vi "Process.vi"(8 "error in":errorcluster, 11 "Logger":refnum<class "Logger.DSC.lvclass">) -> (0 "error out":errorcluster, 3 "Logger out":refnum<class "Logger.DSC.lvclass">)   [LabVIEW 2016, in "Logger.DSC.lvclass"]
doc: "---------------------------------------------------------------\nJKI State Machine Objects™\nhttp://jki.net/state-machine-objects/\nCopyright (C) 2005-2015, JKI <info@jki.net>\nALL RIGHTS RESERVED"
uses:
  Logger.DSC.lvclass
  C:/Program Files (x86)/National Instruments/LabVIEW 2016/vi.lib/JKI/JKI SMO/SMO/SMO.lvclass
  <vilib>/JKI/JKI SMO/SMO/Typedefs/Parent Call--Enum.ctl
  <vilib>/JKI/JKI SMO/SMO/SMO.lvclass
  <resource>/objmgr/ni.var.rc
panel:
  out "Writable":bool
  out "URL":string
  out "Readable":bool
  out "Parent":refnum<k21>
  out "Name":string
  out "Engine":refnum<k21>
  out "Class Identifier":string
  # "For instructions on how to use the JKI State Machine Objects, examples and video tutorials, visit:\nhttp://jki.net/state-machine-objects/\n\nJKI State Machine Objects™\nhttp://jki.net/state-machine-objects/\nCopyright (C) 2005-2015, JKI <info@jki.net>\nALL RIGHTS RESERVED"
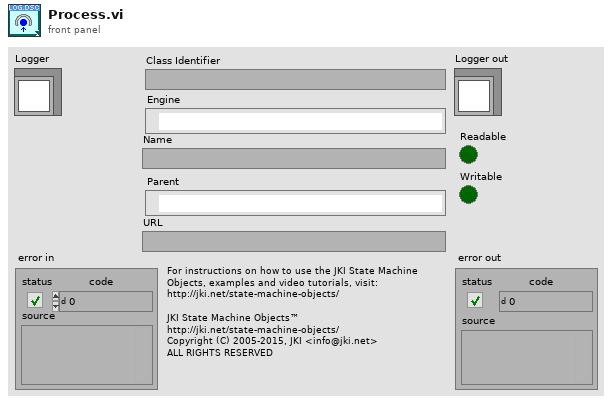
[diagram p1: front panel]
types:
  T1 = typedef "SMO.lvclass/Parent Call--Enum.ctl" = enum16{"Allows parent to run", "Does not request parent to run"}
  T2 = enum32{"invalid app kind", "Development System", "Run Time System", "Student Edition", "Embedded LabVIEW", "Evaluation", "Custom"}
  T3 = enum32{"Invalid", "Standard", "Closed", "Hidden", "Minimized", "Maximized"}
  T4 = enum32{"Bad", "Idle", "Run top level", "Running"}
  T5 = cluster{"Core":cluster{"Current VI Reference":refnum<vi>, "Close Panel on Exit?":bool, "error":errorcluster}, "Self Reference":refnum<class "Logger.DSC.lvclass">, "shared variable address":string, "data in":variant, "data out":variant}
  T6 = cluster{"Current VI Reference":refnum<vi>, "Close Panel on Exit?":bool, "error":errorcluster}
  T7 = typedef "SMO.lvclass/Protected Events.ctl" = cluster{"StopProcesses":refnum<user-event>, "AbortProcesses":refnum<user-event>, "Config Changed":refnum<user-event>, "Dependency":refnum<user-event>}
  T8 = typedef "Logger.DSC.lvclass/PrivateEvents--Cluster.ctl" = cluster{"Set Address":refnum<user-event>, "Write Variable":refnum<user-event>}
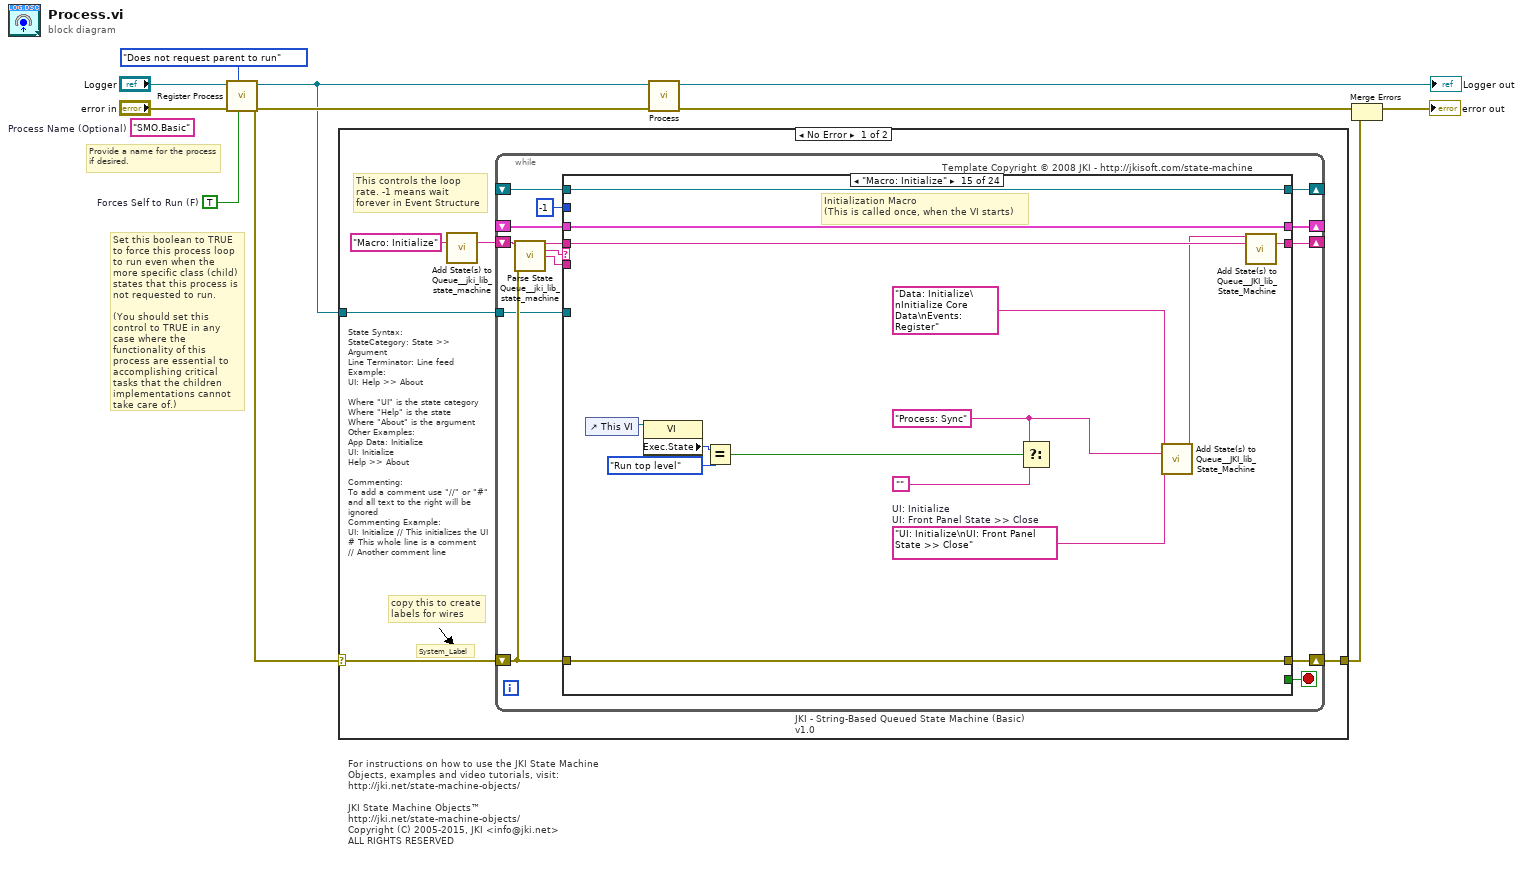
[diagram p0: block diagram]
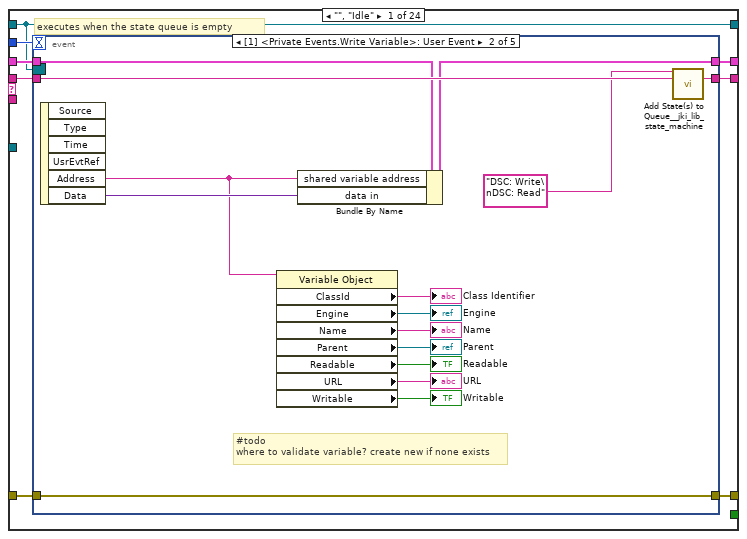
[diagram p2: hidden frame]
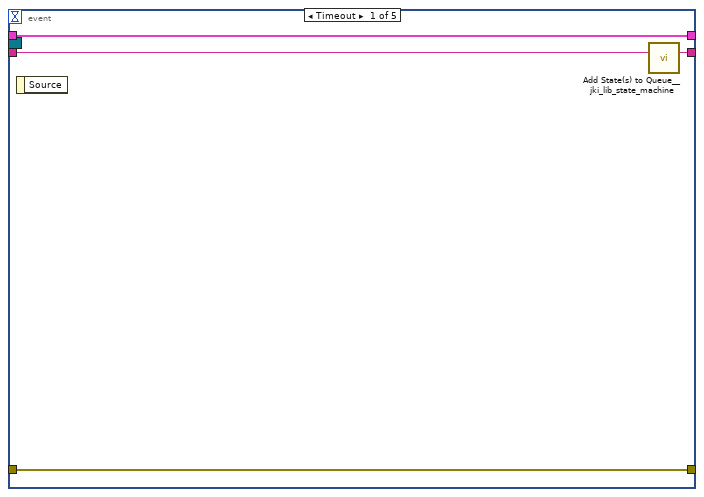
[diagram p3: hidden frame]
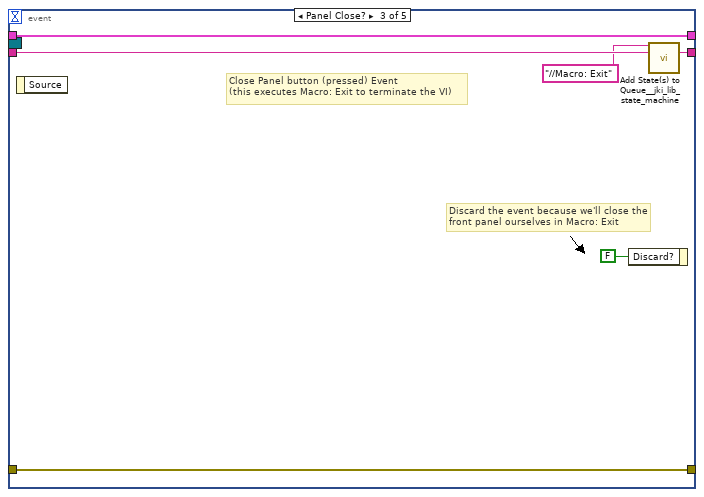
[diagram p4: hidden frame]
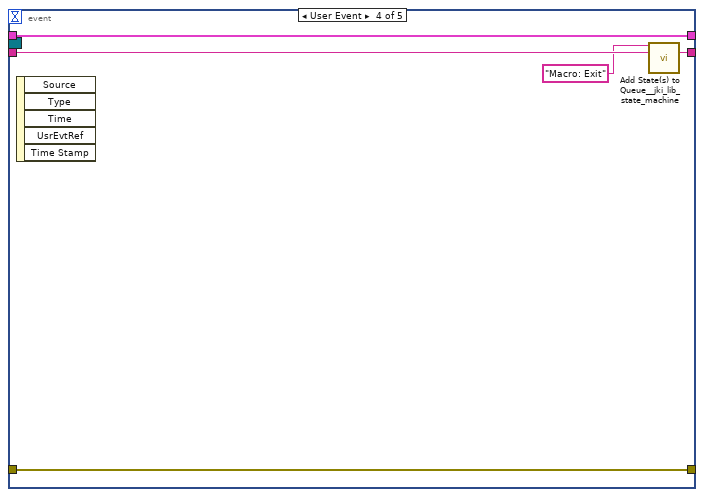
[diagram p5: hidden frame]
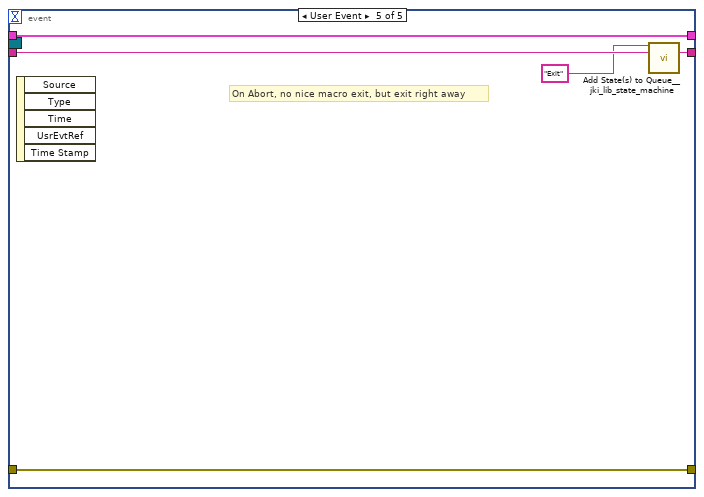
[diagram p6: hidden frame]
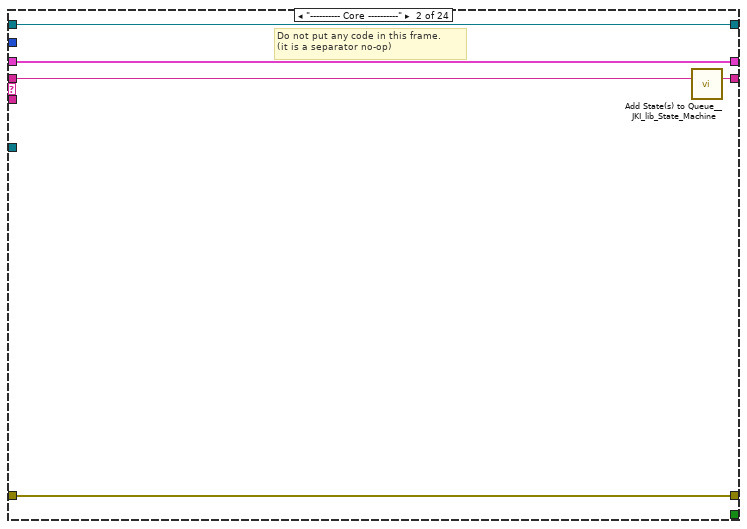
[diagram p7: hidden frame]
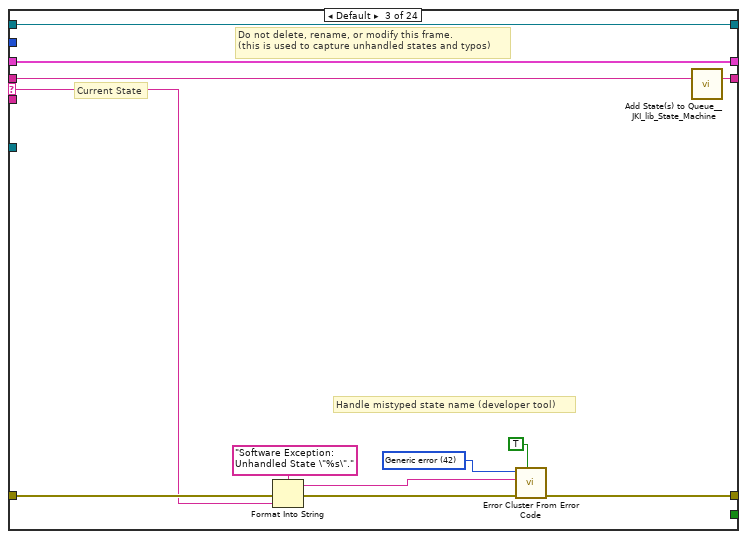
[diagram p8: hidden frame]
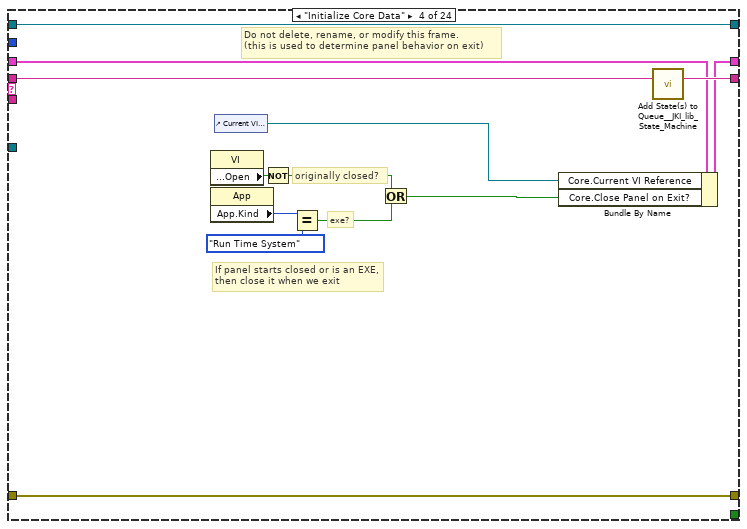
[diagram p9: hidden frame]
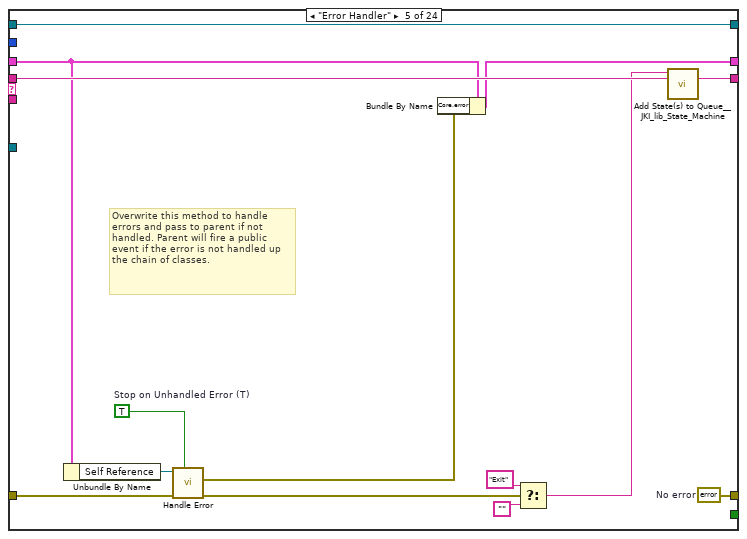
[diagram p10: hidden frame]
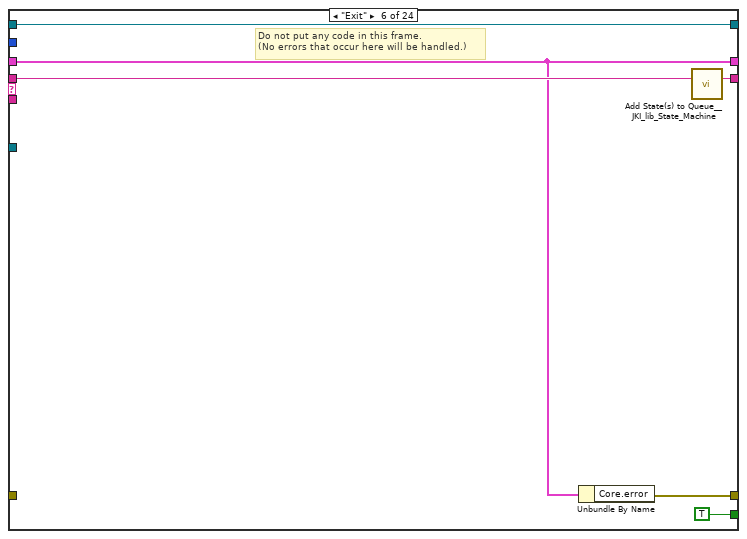
[diagram p11: hidden frame]
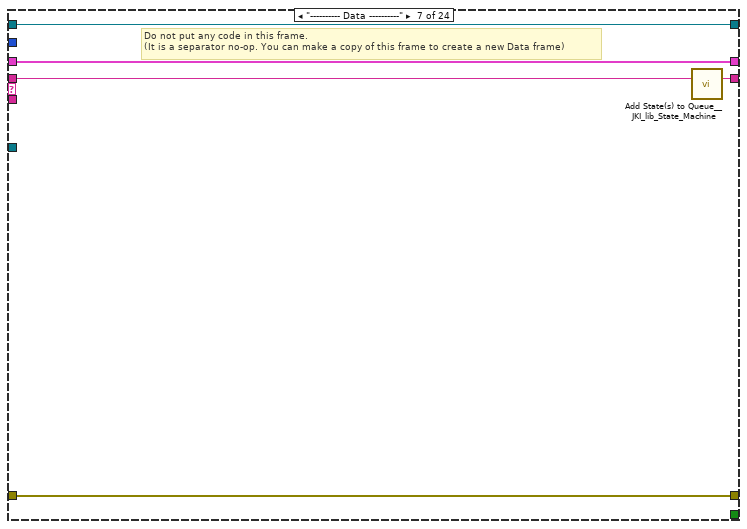
[diagram p12: hidden frame]
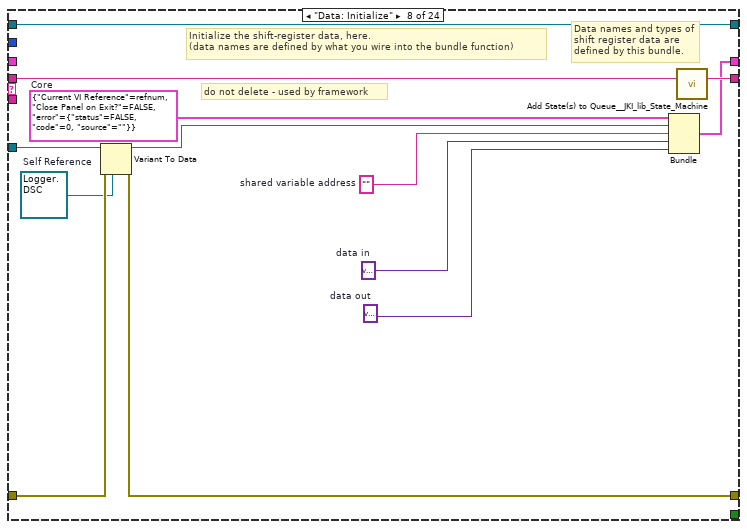
[diagram p13: hidden frame]
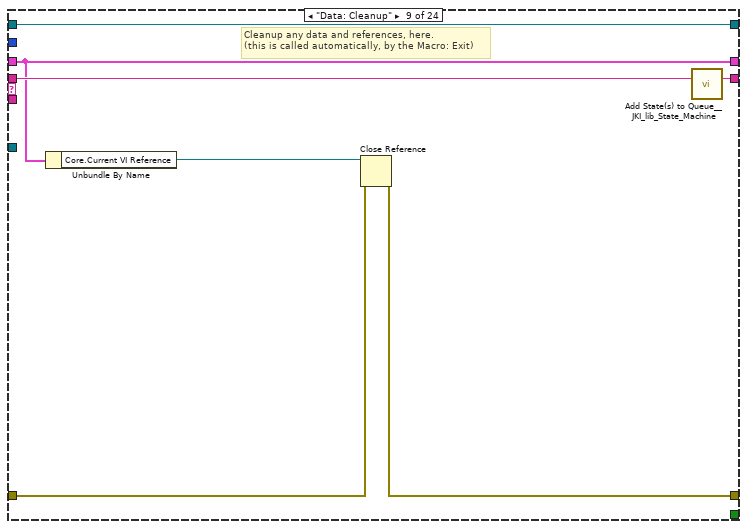
[diagram p14: hidden frame]
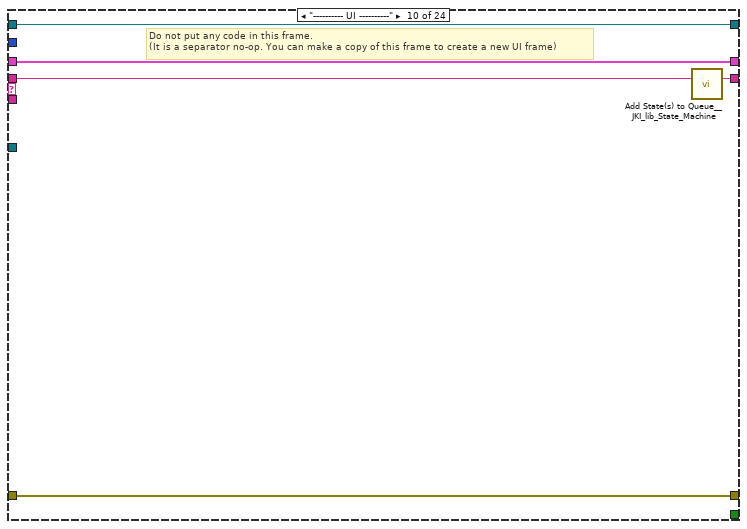
[diagram p15: hidden frame]
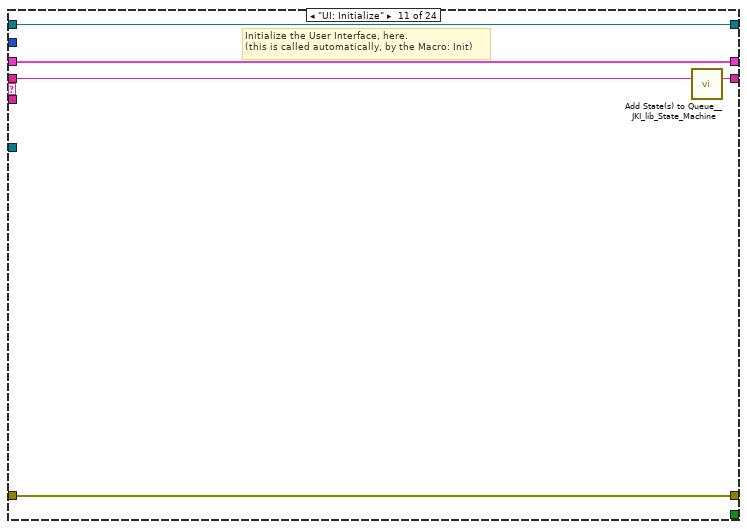
[diagram p16: hidden frame]
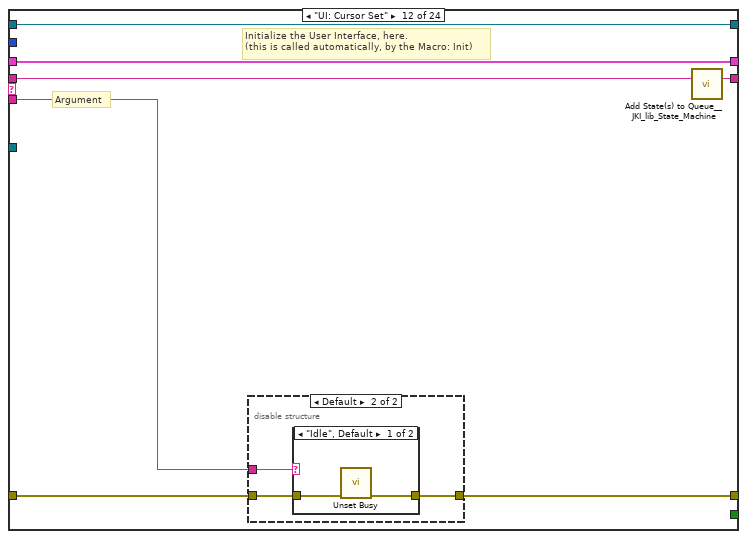
[diagram p17: hidden frame]
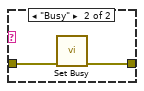
[diagram p19: hidden frame]
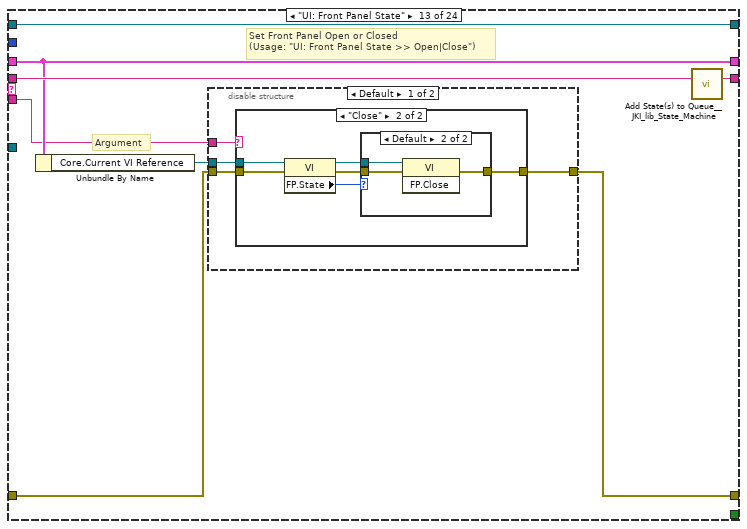
[diagram p20: hidden frame]
diagram:
  w1 = TRUE  # Forces Self to Run (F)
  (unwired) "SMO.Basic"  # Process Name (Optional)
  # "Provide a name for the process\nif desired."
  # "Set this boolean to TRUE to force this process loop to run even when the more specific class (child) states that this process is not requested to run.\n\n(You should set this control to TRUE in any case where the functionality of this process are essential to accomplishing critical tasks that the children implementations cannot take care of.)"
  # "For instructions on how to use the JKI State Machine Objects, examples and video tutorials, visit:\nhttp://jki.net/state-machine-objects/\n\nJKI State Machine Objects™\nhttp://jki.net/state-machine-objects/\nCopyright (C) 2005-2015, JKI <info@jki.net>\nALL RIGHTS RESERVED"
  n1 = call <vilib>:"Register Process.vi"("Forces Self to Run (F)"=w1, "Parent Call"=Parent_Call--Enum."Does not request parent to run", "error in (no error)"="error in", "SMO"="Logger") -> ("error out"=w7:errorcluster, "SMO out"=w6:refnum<class "Logger.DSC.lvclass">)  [unwired: 6 in]
  n2 = case shown="No Error" w7 {
    selector: w7 -> [w12 w308]
    tunnel: w6 -> [w13 _]
    tunnel: [w11 w308] -> w3
    frame No Error {
      # "State Syntax:\nStateCategory: State >> Argument\nLine Terminator: Line feed\nExample:\nUI: Help >> About\n\nWhere \"UI\" is the state category\nWhere \"Help\" is the state\nWhere \"About\" is the argument\nOther Examples:\nApp Data: Initialize\nUI: Initialize\nHelp >> About\n\nCommenting:\nTo add a comment use \"//\" or \"#\" and all text to the right will be ignored\nCommenting Example:\nUI: Initialize // This initializes the UI\n# This whole line is a comment\n// Another comment line"
      # "copy this to create labels for wires"
      # "This controls the loop rate. -1 means wait forever in Event Structure"
      # "System_Label"
      n3 = call <vilib>:"Add State(s) to Queue__jki_lib_state_machine.vi"("State(s) in (\"\")"="Macro: Initialize") -> ("States Out"=w15:string)  [unwired: 14 in]
      n4 = while "JKI - String-Based Queued State Machine (Basic) v1.0" {
        shift-right: [w22] -> _
        shift-left: _ -> [w21]
        shift-right: [w25] -> w11
        shift-left: w12 -> [w19]
        shift-right: [w24] -> _
        shift-left: w15 -> [w26]
        tunnel: w13 -> [w18]
        shift-right: [w17] -> _
        shift-left: _ -> [w16]
        stop <- w23 stop-if-true
        # "Template Copyright © 2008 JKI - http://jkisoft.com/state-machine"
        n5 = call <vilib>:"Parse State Queue__jki_lib_state_machine.vi"("State Queue"=w26, "Error In (no error)"=w19) -> ("Remaining States"=w28:string, "Current State"=w29:string, "Arguments"=w27:string)  [unwired: 11 in]
        n6 = case shown="\"Macro: Initialize\"" w29 {
          selector: w29 -> [_ _ w79 _ _ _ _ _ _ _ _ _ _ _ _ _ _ _ _ _ _ _ _ _]
          tunnel: w28 -> [w37 w77 w83 w102 w116 w122 w127 w140 w147 w152 w157 w164 w180 w212 w226 w240 w245 w256 w261 w274 w280 w285 w295 w307]
          tunnel: w27 -> [_ _ _ _ _ _ _ _ _ _ _ w158 w174 _ _ _ _ _ _ _ _ _ _ _]
          tunnel: w21 -> [w35 w74 w81 w93 w110 w118 w124 _ w142 w149 w155 w162 w176 w209 w222 w231 w242 w253 w258 w272 w278 w283 w291 w302]
          tunnel: [w34 w75 w85 w99 w111 w117 w125 w136 w143 w150 w154 w159 w177 w210 w224 w238 w243 w247 w259 w267 w276 w281 w292 w297] -> w25
          tunnel: w19 -> [w33 w75 w84 w99 w112 _ w125 w137 w144 w150 w154 w160 w178 w210 w224 w238 w243 w248 w259 w268 w276 w281 w287 w298]
          tunnel: [w36 w76 w82 w101 w115 w121 w126 w139 w146 w151 w156 w163 w179 w211 w225 w239 w244 w255 w260 w273 w279 w284 w294 w306] -> w24
          tunnel: [_ _ _ _ _ TRUE _ _ _ _ _ _ _ _ _ _ _ _ _ _ _ _ _ _] -> w23
          tunnel: [w32 w74 w81 w100 w109 w118 w124 w138 w142 w149 w155 w162 w176 w209 w222 w231 w242 w253 w258 w272 w278 w283 w291 w302] -> w22
          tunnel: -1 ("Timeout") -> [w31 _ _ _ _ _ _ _ _ _ _ _ _ _ _ _ _ _ _ _ _ _ _ _]
          tunnel: w18 -> [_ _ _ _ _ _ _ w134 _ _ _ _ _ _ _ _ _ _ _ _ _ _ _ _]
          tunnel: [w30 w73 w78 w90 w114 w119 w123 w132 w141 w148 w153 w161 w173 w208 w223 w232 w241 w254 w257 w271 w277 w282 w293 w305] -> w17
          tunnel: w16 -> [w30 w73 w78 w90 w114 w119 w123 w132 w141 w148 w153 w161 w173 w208 w223 w232 w241 w254 w257 _ w277 w282 w293 w305]
          frame "", "Idle" {
            # "executes when the state queue is empty"
            n7 = event shown="[1] <Private Events.Write Variable>: User Event" {
              selector: w30 -> [_ _ _ _ _]
              dyn-events: _ -> [_ _ _ _ _]
              timeout: w31 -> [_ _ _ _ _]
              tunnel: w37 -> [w41 w56 w62 w67 w72]
              tunnel: [w40 w55 w61 w66 w71] -> w36
              tunnel: w35 -> [w39 w53 w59 w64 w69]
              tunnel: [w38 w54 w60 w65 w70] -> w34
              tunnel: w33 -> [w38 w54 w60 w65 w70]
              tunnel: [w39 w52 w59 w64 w69] -> w32
              event Timeout {
                n8 = event-data() -> ()  [unwired: 1 in, 1 out]
                n9 = call <vilib>:"Add State(s) to Queue__jki_lib_state_machine.vi"("State(s) in (\"\")"=w41) -> ("States Out"=w40:string)  [unwired: 14 in]
              }
              event User Event {
                # "#todo\nwhere to validate variable? create new if none exists"
                n10 = event-data() -> ("Address"=w42:string, "Data"=w50:variant)  [unwired: 1 in, 4 out]
                n11 = property class="Variable Object"(reference=w42) -> ("ClassId"=→"Class Identifier":string, "Engine"=→"Engine":refnum<k21>, "Name"=→"Name":string, "Parent"=→"Parent":refnum<k21>, "Readable"=→"Readable":bool, "URL"=→"URL":string, "Writable"=→"Writable":bool)  [unwired: 1 in, 2 out]
                n12 = Bundle By Name(cluster=w53, "shared variable address"=w42, "data in"=w50) -> (w52:T5)
                n13 = call <vilib>:"Add State(s) to Queue__jki_lib_state_machine.vi"("State(s) in Front (\"\")"="DSC: Write\nDSC: Read" ("State(s) in Front (\"\")"), "State(s) in (\"\")"=w56) -> ("States Out"=w55:string)  [unwired: 13 in]
              }
              event Panel Close? {
                # "Discard the event because we'll close the front panel ourselves in Macro: Exit"
                # "Close Panel button (pressed) Event\n(this executes Macro: Exit to terminate the VI)"
                n14 = event-data() -> ()  [unwired: 1 in, 1 out]
                n15 = event-data("Discard?"=FALSE) -> ()  [unwired: 1 in, 1 out]
                n16 = call <vilib>:"Add State(s) to Queue__jki_lib_state_machine.vi"("State(s) in Front (\"\")"="//Macro: Exit", "State(s) in (\"\")"=w62) -> ("States Out"=w61:string)  [unwired: 13 in]
              }
              event User Event {
                n17 = event-data() -> ()  [unwired: 1 in, 5 out]
                n18 = call <vilib>:"Add State(s) to Queue__jki_lib_state_machine.vi"("State(s) in Front (\"\")"="Macro: Exit", "State(s) in (\"\")"=w67) -> ("States Out"=w66:string)  [unwired: 13 in]
              }
              event User Event {
                # "On Abort, no nice macro exit, but exit right away"
                n19 = event-data() -> ()  [unwired: 1 in, 5 out]
                n20 = call <vilib>:"Add State(s) to Queue__jki_lib_state_machine.vi"("State(s) in Front (\"\")"="Exit", "State(s) in (\"\")"=w72) -> ("States Out"=w71:string)  [unwired: 13 in]
              }
            }
          }
          frame "---------- Core ----------" {
            # "Do not put any code in this frame.\n(it is a separator no-op)"
            n21 = call <vilib>:"Add State(s) to Queue__JKI_lib_State_Machine.vi"("State(s) in (\"\")"=w77) -> ("States Out"=w76:string)  [unwired: 14 in]
          }
          frame Default {
            w88 = 42 items=["No error", "Argument error", "Memory is full", "Out of zone", "End of file", "File already open", "Generic file I/O error", "File not found", "File permission error", "Disk is full", "Duplicate path", "Too many files open", "System feature not enabled", "Resource file not found", "Cannot add resource", "Resource not found", "Image not found", "Image memory error", "Pen does not exist", "Config type invalid", "Config token not found", "Config parse error", "Config memory error", "Bad external code format", "Bad external code offset", "External code not present", "Null window", "Destroy window error", "Null menu", "Print aborted", "Bad print record", "Print driver error", "Windows error during printing", "Memory error during printing", "Print dialog error", "Generic print error", "Invalid device refnum", "Device not found", "Device parameter error", "Device unit error", "Cannot open device", "Device call aborted", "Generic error", "Cancelled by user", "Object ID too low", "Object ID too high", "Object not in heap", "Unknown heap", "Unknown object (invalid DefProc)", "Unknown object (DefProc not in table)", "Message out of range", "Invalid (null) method", "Unknown message", "Manager call not supported", "Bad address", "Network operation in progress", "Network operation timed out", "Connection is busy", "Network attribute not supported", "Network error", "Address in use", "System out of memory", "Connection aborted", "Connection refused", "Not connected", "Already connected", "Connection closed", "Initialization error (interapplication manager)", "Bad occurrence", "Wait on unbound occurrence handler", "Occurrence queue overflow", "Datalog type conflict", "Unused", "Unrecognized type (interapplication manager)", "Memory corrupt", "Failed to make temporary DLL", "Old CIN version", "Drag socket not found", "Failed to load drop-object", "Failed to register OLE object", "Failed to release OLE object", "Format specifier type mismatch", "Unknown format specifier", "Too few format specifiers", "Too many format specifiers", "Scan failed", "Newer CIN version", "Error converting to variant", "Runtime menu error", "Password tampered", "Variant attribute not found", "Incompatible variant data type", "Event data is not available", "Event Store is not present", "Occurrence is not found", "Event Queue is not created", "Event info is not available", "Refnum passed is NULL", "Error retrieving Class GUID", "Error retrieving CoClass GUID", "Error retrieving TypeLib GUID.", "Bad built application magic bytes.", "Specific driver is different from the specific driver associated with the Logical Name.", "There is no session opened to the class driver.", "Max Error", "MAX - Error with config objects", "MAX - Error loading configuration", "MAX - Group not supported"]
            # "Current State"
            # "Do not delete, rename, or modify this frame.\n(this is used to capture unhandled states and typos)"
            # "Handle mistyped state name (developer tool)"
            n22 = Format Into String(format string="Software Exception: Unhandled State \"%s\"." ("message"), error in=w84, w79) -> (resulting string=w87:string, error out=w86:errorcluster)  [unwired: 1 in]
            n23 = call <vilib>:"Error Cluster From Error Code.vi"("show call chain? (False)"=TRUE, "error in (no error)"=w86, "error message (\"\")"=w87, "error code (0)"=w88) -> ("error out"=w85:errorcluster)  [unwired: 5 in]
            n24 = call <vilib>:"Add State(s) to Queue__JKI_lib_State_Machine.vi"("State(s) in (\"\")"=w83) -> ("States Out"=w82:string)  [unwired: 14 in]
          }
          frame "Initialize Core Data" {
            # "Do not delete, rename, or modify this frame.\n(this is used to determine panel behavior on exit)"
            # "originally closed?"
            # "exe?"
            # "If panel starts closed or is an EXE, then close it when we exit"
            n25 = property class="VI"() -> ("Front Panel.Open"=w98:bool)  [unwired: 2 in, 2 out]
            n26 = property class="App"() -> ("App.Kind"=w97:T2)  [unwired: 2 in, 2 out]
            n27 = control-ref of="Current VI Reference"() -> (w91:refnum<vi>)
            n28 = Not(x=w98) -> (.not. x?=w95:bool)
            n29 = Equal?(x=w97, y=T2."Run Time System" ("Application:Kind")) -> (x = y?=w94:bool)
            n30 = Or(x=w95, y=w94) -> (x .or. y?=w92:bool)
            n31 = Bundle By Name(cluster=w93, "Core.Current VI Reference"=w91, "Core.Close Panel on Exit?"=w92) -> (w100:T5)
            n32 = call <vilib>:"Add State(s) to Queue__JKI_lib_State_Machine.vi"("State(s) in (\"\")"=w102) -> ("States Out"=w101:string)  [unwired: 14 in]
          }
          frame "Error Handler" {
            w103 = TRUE  # Stop on Unhandled Error (T)
            w111 = errorcluster {"status"=FALSE, "code"=0, "source"=""}  # No error
            # "Overwrite this method to handle errors and pass to parent if not handled. Parent will fire a public event if the error is not handled up the chain of classes."
            n33 = Unbundle By Name(w110) -> ("Self Reference"=w113:refnum<class "Logger.DSC.lvclass">)
            n34 = call-dynamic "Handle Error.vi"("Stop on Unhandled Error (T)"=w103, "error in"=w112, "SMO"=w113) -> ("handling error"=w104:errorcluster, "Unhandled error"=w107:errorcluster)  [unwired: 6 in, 1 out]
            n35 = Bundle By Name(cluster=w110, "Core.error"=w107) -> (w109:T5)
            n36 = Select(t="Exit", s=w104, f="") -> (s? t:f=w108:string)
            n37 = call <vilib>:"Add State(s) to Queue__JKI_lib_State_Machine.vi"("State(s) in Front (\"\")"=w108, "State(s) in (\"\")"=w116) -> ("States Out"=w115:string)  [unwired: 13 in]
          }
          frame "Exit" {
            # "Do not put any code in this frame.\n(No errors that occur here will be handled.)"
            n38 = Unbundle By Name(w118) -> ("Core.error"=w117:errorcluster)
            n39 = call <vilib>:"Add State(s) to Queue__JKI_lib_State_Machine.vi"("State(s) in (\"\")"=w122) -> ("States Out"=w121:string)  [unwired: 14 in]
          }
          frame "---------- Data ----------" {
            # "Do not put any code in this frame.\n(It is a separator no-op. You can make a copy of this frame to create a new Data frame)"
            n40 = call <vilib>:"Add State(s) to Queue__JKI_lib_State_Machine.vi"("State(s) in (\"\")"=w127) -> ("States Out"=w126:string)  [unwired: 14 in]
          }
          frame "Data: Initialize" {
            w128 = variant  # data out
            w129 = variant  # data in
            w130 = ""  # shared variable address
            w131 = T6 {"Current VI Reference"=refnum, "Close Panel on Exit?"=FALSE, "error"={"status"=FALSE, "code"=0, "source"=""}}  # Core
            w135 = refnum<class "Logger.DSC.lvclass"> refnum  # Self Reference
            # "do not delete - used by framework"
            # "Data names and types of shift register data are defined by this bundle."
            # "Initialize the shift-register data, here.\n(data names are defined by what you wire into the bundle function)"
            n41 = Variant To Data(error in=w137, type=w135, Variant=w134) -> (data=w133:refnum<class "Logger.DSC.lvclass">, error out=w136:errorcluster)
            n42 = Bundle("Core"=w131, "Self Reference"=w133, "shared variable address"=w130, "data in"=w129, "data out"=w128) -> (w138:T5)  [unwired: 1 in]
            n43 = call <vilib>:"Add State(s) to Queue__JKI_lib_State_Machine.vi"("State(s) in (\"\")"=w140) -> ("States Out"=w139:string)  [unwired: 14 in]
          }
          frame "Data: Cleanup" {
            # "Cleanup any data and references, here.\n(this is called automatically, by the Macro: Exit)"
            n44 = Unbundle By Name(w142) -> ("Core.Current VI Reference"=w145:refnum<vi>)
            n45 = Close Reference(reference=w145, error in (no error)=w144) -> (error out=w143:errorcluster)
            n46 = call <vilib>:"Add State(s) to Queue__JKI_lib_State_Machine.vi"("State(s) in (\"\")"=w147) -> ("States Out"=w146:string)  [unwired: 14 in]
          }
          frame "---------- UI ----------" {
            # "Do not put any code in this frame.\n(It is a separator no-op. You can make a copy of this frame to create a new UI frame)"
            n47 = call <vilib>:"Add State(s) to Queue__JKI_lib_State_Machine.vi"("State(s) in (\"\")"=w152) -> ("States Out"=w151:string)  [unwired: 14 in]
          }
          frame "UI: Initialize" {
            # "Initialize the User Interface, here.\n(this is called automatically, by the Macro: Init)"
            n48 = call <vilib>:"Add State(s) to Queue__JKI_lib_State_Machine.vi"("State(s) in (\"\")"=w157) -> ("States Out"=w156:string)  [unwired: 14 in]
          }
          frame "UI: Cursor Set" {
            # "Argument"
            # "Initialize the User Interface, here.\n(this is called automatically, by the Macro: Init)"
            n49 = disable-structure shown="Default" {
              disable-tunnel: w160 -> [w165 w168]
              disable-tunnel: [w165 w167] -> w159
              disable-tunnel: w158 -> [_ w166]
              frame condition #0 {
              }
              frame condition #1 (active) {
                n50 = case shown="\"Idle\", Default" w166 {
                  tunnel: w168 -> [w170 w172]
                  tunnel: [w169 w171] -> w167
                  frame "Idle", Default {
                    n51 = call <vilib>:"Unset Busy.vi"("error in (no error)"=w170) -> ("error out"=w169:errorcluster)  [unwired: 10 in]
                  }
                  frame "Busy" {
                    n52 = call <vilib>:"Set Busy.vi"("error in (no error)"=w172) -> ("error out"=w171:errorcluster)  [unwired: 9 in, 1 out]
                  }
                }
              }
            }
            n53 = call <vilib>:"Add State(s) to Queue__JKI_lib_State_Machine.vi"("State(s) in (\"\")"=w164) -> ("States Out"=w163:string)  [unwired: 14 in]
          }
          frame "UI: Front Panel State" {
            # "Argument"
            # "Set Front Panel Open or Closed\n(Usage: \"UI: Front Panel State >> Open|Close\")"
            n54 = Unbundle By Name(w176) -> ("Core.Current VI Reference"=w175:refnum<vi>)
            n55 = disable-structure shown="Default" {
              disable-tunnel: w178 -> [w184 w207]
              disable-tunnel: [w183 w207] -> w177
              disable-tunnel: w175 -> [w182 _]
              disable-tunnel: w174 -> [w181 _]
              frame condition #0 (active) {
                n56 = case shown="\"Close\"" w181 {
                  tunnel: w184 -> [w188 w201]
                  tunnel: [w190 w202] -> w183
                  tunnel: w182 -> [w189 w199]
                  frame "Open", Default {
                    n57 = property class="VI"(reference=w189, error in=w188) -> (reference out=w186:refnum<vi>, error out=w187:errorcluster, "FP.State"=w185:T3)
                    n58 = case shown="\"Closed\"" w185 {
                      tunnel: [w193 w196] -> w190
                      tunnel: w187 -> [w192 w196]
                      tunnel: w186 -> [w191 _]
                      frame "Closed" {
                        n59 = invoke class="VI" method="FP.Open"(reference=w191, error in=w192, "Activate"=TRUE, "State"=T3."Standard") -> (error out=w193:errorcluster)  [unwired: 1 in, 4 out]
                      }
                      frame Default {
                      }
                    }
                  }
                  frame "Close" {
                    n60 = property class="VI"(reference=w199, error in=w201) -> (reference out=w198:refnum<vi>, error out=w200:errorcluster, "FP.State"=w197:T3)
                    n61 = case shown="Default" w197 {
                      tunnel: [w203 w206] -> w202
                      tunnel: w200 -> [w203 w205]
                      tunnel: w198 -> [_ w204]
                      frame "Invalid", "Closed" {
                      }
                      frame Default {
                        n62 = invoke class="VI" method="FP.Close"(reference=w204, error in=w205) -> (error out=w206:errorcluster)  [unwired: 1 in, 2 out]
                      }
                    }
                  }
                }
              }
              frame condition #1 {
              }
            }
            n63 = call <vilib>:"Add State(s) to Queue__JKI_lib_State_Machine.vi"("State(s) in (\"\")"=w180) -> ("States Out"=w179:string)  [unwired: 14 in]
          }
          frame "---------- Macro ----------" {
            # "Do not put any code in this frame.\n(It is a separator no-op. You can make a copy of this frame to create a new Macro frame)"
            n64 = call <vilib>:"Add State(s) to Queue__JKI_lib_State_Machine.vi"("State(s) in (\"\")"=w212) -> ("States Out"=w211:string)  [unwired: 14 in]
          }
          frame "Macro: Initialize" {
            w217 = "UI: Initialize\nUI: Front Panel State >> Close"  # UI: Initialize UI: Front Panel State >> Close
            w213 = "Process: Sync"
            # "Initialization Macro\n(This is called once, when the VI starts)"
            n65 = control-ref of="This VI"() -> (w215:refnum<vi>)
            n66 = property class="VI"(reference=w215) -> ("Exec.State"=w214:T4)  [unwired: 1 in, 2 out]
            n67 = Equal?(x=w214, y=T4."Run top level") -> (x = y?=w220:bool)
            n68 = Select(t=w213, s=w220, f="") -> ()  [unwired: 1 out]
            n69 = call <vilib>:"Add State(s) to Queue__JKI_lib_State_Machine.vi"("State(s) in Front (\"\")"="Data: Initialize\nInitialize Core Data\nEvents: Register", "State(s) in (\"\")"=w213, "State(s) at Back (\"\")"=w217) -> ("States Out"=w216:string)  [unwired: 12 in]
            n70 = call <vilib>:"Add State(s) to Queue__JKI_lib_State_Machine.vi"("State(s) in Front (\"\")"=w216, "State(s) in (\"\")"=w226) -> ("States Out"=w225:string)  [unwired: 13 in]
          }
          frame "Macro: Exit" {
            w236 = "UI: Front Panel State >> Close"  # UI: Front Panel State >> Close
            # "Exit Macro\n(This is called once, when the VI exits)"
            n71 = Unbundle By Name(w231) -> ("Core.Close Panel on Exit?"=w237:bool)
            n72 = Select(t=w236, s=w237, f="") -> (s? t:f=w234:string)
            n73 = call <vilib>:"Add State(s) to Queue__JKI_lib_State_Machine.vi"("State(s) in Front (\"\")"="Data: Cleanup\nEvents: Unregister", "State(s) in (\"\")"="Process: Sync", "State(s) at Back (\"\")"="Exit") -> ("States Out"=w228:string)  [unwired: 12 in]
            n74 = call <vilib>:"Add State(s) to Queue__JKI_lib_State_Machine.vi"("State(s) in (\"\")"=w234, "State(s) at Back (\"\")"=w228) -> ("States Out"=w233:string)  [unwired: 13 in]
            n75 = call <vilib>:"Add State(s) to Queue__JKI_lib_State_Machine.vi"("State(s) in Front (\"\")"=w233, "State(s) in (\"\")"=w240) -> ("States Out"=w239:string)  [unwired: 13 in]
          }
          frame "---------- Process ----------" {
            # "Template Separator\n(You can make a copy of, or modify, this frame)"
            n76 = call <vilib>:"Add State(s) to Queue__JKI_lib_State_Machine.vi"("State(s) in (\"\")"=w245) -> ("States Out"=w244:string)  [unwired: 14 in]
          }
          frame "Process: Sync" {
            n77 = Unbundle By Name(w253) -> ("Self Reference"=w249:refnum<class "Logger.DSC.lvclass">)
            n78 = call <vilib>:"WaitOnProcessSync.vi"("error in (no error)"=w248, "SMO"=w249) -> ("error out"=w247:errorcluster, "Don't run?"=w252:bool)  [unwired: 7 in, 1 out]
            n79 = Select(t="Data: Cleanup\nEvents: Unregister\nExit", s=w252, f="") -> (s? t:f=w246:string)
            n80 = call <vilib>:"Add State(s) to Queue__JKI_lib_State_Machine.vi"("State(s) in Front (\"\")"=w246, "State(s) in (\"\")"=w256) -> ("States Out"=w255:string)  [unwired: 13 in]
          }
          frame "---------- Events ----------" {
            # "Template Separator\n(You can make a copy of, or modify, this frame)"
            n81 = call <vilib>:"Add State(s) to Queue__JKI_lib_State_Machine.vi"("State(s) in (\"\")"=w261) -> ("States Out"=w260:string)  [unwired: 14 in]
          }
          frame "Events: Register" {
            # "Expand to add\nmore events"
            n82 = Unbundle By Name(w272) -> ("Self Reference"=w269:refnum<class "Logger.DSC.lvclass">)
            n83 = call <vilib>:"GetProtectedEvents.vi"("SMO"=w269) -> ("error out"=w265:errorcluster, "SMO Protected Events"=w270:T7, "SMO out"=w264:refnum<class "Logger.DSC.lvclass">)  [unwired: 8 in]
            n84 = call "Logger.GetPrivateEvents.vi"("Logger"=w264) -> ("error out"=w262:errorcluster, "Private Events"=w263:T8)  [unwired: 8 in, 1 out]
            n85 = register-events(w270, w263) -> (reference out=w271:refnum<event-registration>, error out=w266:errorcluster)  [unwired: 2 in]
            n86 = Merge Errors(w262, w268, w266, w265) -> (w267:errorcluster)
            n87 = call <vilib>:"Add State(s) to Queue__JKI_lib_State_Machine.vi"("State(s) in (\"\")"=w274) -> ("States Out"=w273:string)  [unwired: 14 in]
          }
          frame "Events: Unregister" {
            n88 = Unregister For Events(event registration refnum=w277, error in=w276) -> (error out=w275:errorcluster)
            n89 = call <vilib>:"Clear Errors.vi"("error in (no error)"=w275) -> ()  [unwired: 5 in, 2 out]
            n90 = call <vilib>:"Add State(s) to Queue__JKI_lib_State_Machine.vi"("State(s) in (\"\")"=w280) -> ("States Out"=w279:string)  [unwired: 14 in]
          }
          frame "---------- DSC ----------" {
            n91 = call <vilib>:"Add State(s) to Queue__JKI_lib_State_Machine.vi"("State(s) in (\"\")"=w285) -> ("States Out"=w284:string)  [unwired: 14 in]
          }
          frame "DSC: Write" {
            n92 = Unbundle By Name(w291) -> ("shared variable address"=w286:string, "data in"=w290:variant)
            n93 = property class="Variable Object" props=["ClassId", "Engine", "Name", "Parent", "Readable", "URL", "Writable"](reference=w286) -> ()  [unwired: 1 in, 9 out]
            n94 = shared-variable-write(w286, w287, w290) -> (w288:refnum<k21>, w289:errorcluster)
            n95 = Close Variable Connection(8:w289, 11:w288) -> (0:w292:errorcluster)
            n96 = call <vilib>:"Add State(s) to Queue__JKI_lib_State_Machine.vi"("State(s) in (\"\")"=w295) -> ("States Out"=w294:string)  [unwired: 14 in]
          }
          frame "DSC: Read" {
            n97 = Unbundle By Name(w302) -> ("Self Reference"=w296:refnum<class "Logger.DSC.lvclass">, "shared variable address"=w303:string)
            n98 = shared-variable-read(w303, w298, variant) -> (w299:refnum<k21>, w304:errorcluster, w300:variant)  [unwired: 1 out]
            n99 = call "Logger.ReadVariable.vi"("error in (no error)"=w304, "Data"=w300, "Address"=w299, "Logger"=w296) -> ("error out"=w297:errorcluster)  [unwired: 6 in, 1 out]
            n100 = call <vilib>:"Add State(s) to Queue__JKI_lib_State_Machine.vi"("State(s) in (\"\")"=w307) -> ("States Out"=w306:string)  [unwired: 14 in]
          }
        }
      }
    }
    frame Error {
    }
  }
  n101 = call-parent "Process.vi"("error in"=w7, "SMO"=w6) -> ("error out"=w4:errorcluster, "SMO out"=→"Logger out":refnum<class "Logger.DSC.lvclass">)  [unwired: 8 in]
  n102 = Merge Errors(w4, w3) -> (→"error out":errorcluster)
